vi "Get Travel - Force Reading.vi"(8 "error in (no error)":errorcluster, 11 "ESM303 in":refnum<class "ESM303.lvclass">) -> (0 "error out":errorcluster, 1 "Force Reading":dbl format="%.4f", 2 "Travel Reading":dbl format="%.4f", 3 "ESM303 out":refnum<class "ESM303.lvclass">)   [LabVIEW 2018, in "ESM303.lvlib" / "ESM303.lvclass"]
uses:
  ESM303.lvclass
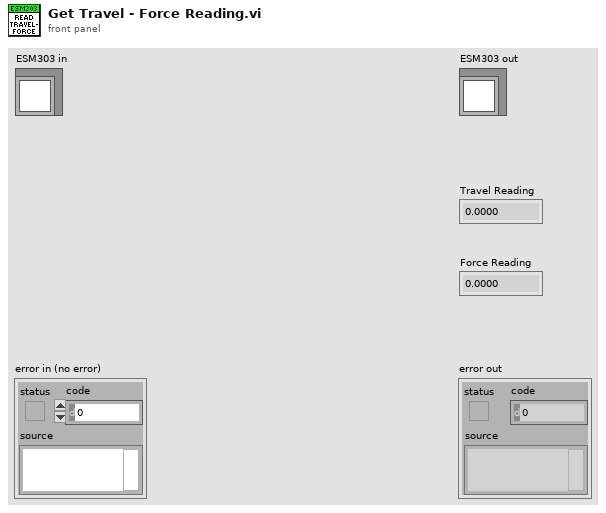
[diagram p1: front panel]
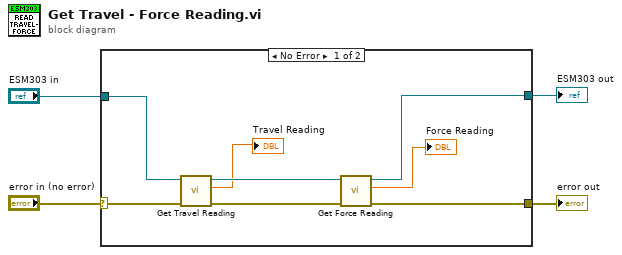
[diagram p0: block diagram]
diagram:
  n1 = case shown="No Error" "error in (no error)" {
    selector: "error in (no error)" -> [w12 w14]
    tunnel: [w5 w14] -> w4
    tunnel: [w6 w13] -> w3
    tunnel: "ESM303 in" -> [w11 w13]
    frame No Error {
      n2 = call-dynamic "Get Travel Reading.vi"("error in (no error)"=w12, "ESM303 in"=w11) -> ("error out"=w9:errorcluster, "Reading"=→"Travel Reading":dbl, "ESM303 out"=w10:refnum<class "ESM303.lvclass">)  [unwired: 7 in]
      n3 = call-dynamic "Get Force Reading.vi"("error in (no error)"=w9, "ESM303 in"=w10) -> ("error out"=w5:errorcluster, "Reading"=→"Force Reading":dbl, "ESM303 out"=w6:refnum<class "ESM303.lvclass">)  [unwired: 7 in]
    }
    frame Error {
    }
  }
  "error out" <- w4
  "ESM303 out" <- w3
